vi "Homing v2.vi"(7 "Robot In":i32, 8 "error in":errorcluster, 9 "ToolInsertionOffset":dbl=-54.76, 10 "ToolType":i32=6, 11 "FPGA VI Reference In":refnum<k20>) -> (0 "error out":errorcluster, 1 "Last Stage Posit":dbl[](array[numeric]), 2 "Last Joint Posit":dbl[](array[numeric]), 3 "FPGA VI Reference Out":refnum<k20>)   [LabVIEW 2016]
uses:
  Subsystems/Global Variables.vi
  <vilib>/platform/TimedLoop/XDataNode/XDataNode.xnode
  <vilib>/Platform/TimedLoop/XDataNode/timing_clust.ctl
  <vilib>/Platform/TimedLoop/XDataNode/XDNodeRunTimeDep.lvlib
  <vilib>/Platform/TimedLoop/XDataNode/wakeup.ctl
  <vilib>/Platform/TimedLoop/XDataNode/nitl_modes.ctl
  <vilib>/rvi/interface/nirviReadWriteControl/nirviReadWriteControl.xnode
  Library/KevinLibraryAll/labview2011/kevLib2011.lvlib
  Library/mjglib/var_OCTzHomeDir.vi
  Functions/EyeRobotDLL.dll
  FPGA Bitfiles/PhantomControlPI_FPGATarget_QuadCtr2_E2412E44.lvbitx
  IRISS_FPGA_IO.vi
  NiFpgaLv.dll
  <vilib>/Utility/error.llb/Error Cluster From Error Code.vi
  <vilib>/rvi/errors/niLvFpgaAdjustHostInterfaceError.vi
panel:
  out "Grasp":dbl
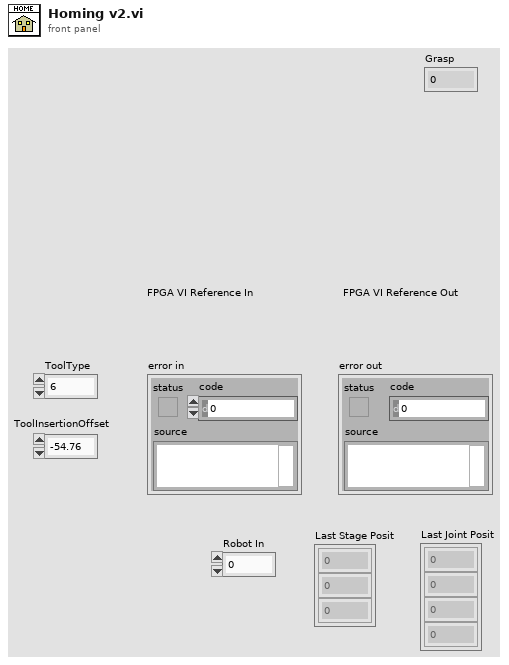
[diagram p1: front panel]
types:
  T1 = typedef "XDNodeRunTimeDep.lvlib/timing_clust.ctl" = cluster{"Expected End [f-1]":u64, "Actual End [f-1]":u64, "Finished Late? [f-1]":bool, "Expected End [i-1]":u64, "Actual End [i-1]":u64, "Finished Late? [i-1]":bool, "Expected Start [i]":u64, "Actual Start [i]":u64, "Expected Start [f]":u64, "Actual Start [f]":u64, "Source Name":string, "Structure Name":string, "Period":i64, "Deadline":i64, "Offset":i64, "Start":i64, "Priority":i32, "Timeout":i32, "Mode":T2, "Wakeup Reason":T3, "Error":errorcluster, "Source Type":string, "Secondary Source Type":string, "Global End Time":u64, "Global Start Time":u64, "Frame Duration":u64, "Iteration Duration":u64, "Assigned CPU":i32, "I/O Scan Engine Mode":u32}
  T2 = typedef "XDNodeRunTimeDep.lvlib/nitl_modes.ctl" = enum32{"No Change", "Process missed periods, maintain original phase", "Discard missed periods, maintain original phase", "Process missed periods, ignore original phase", "Discard missed periods, ignore original phase"}
  T3 = typedef "XDNodeRunTimeDep.lvlib/wakeup.ctl" = enum32{"Normal", "Aborted", "Asynchronous wakeup", "Timing source error", "Timed loop error", "Timeout"}
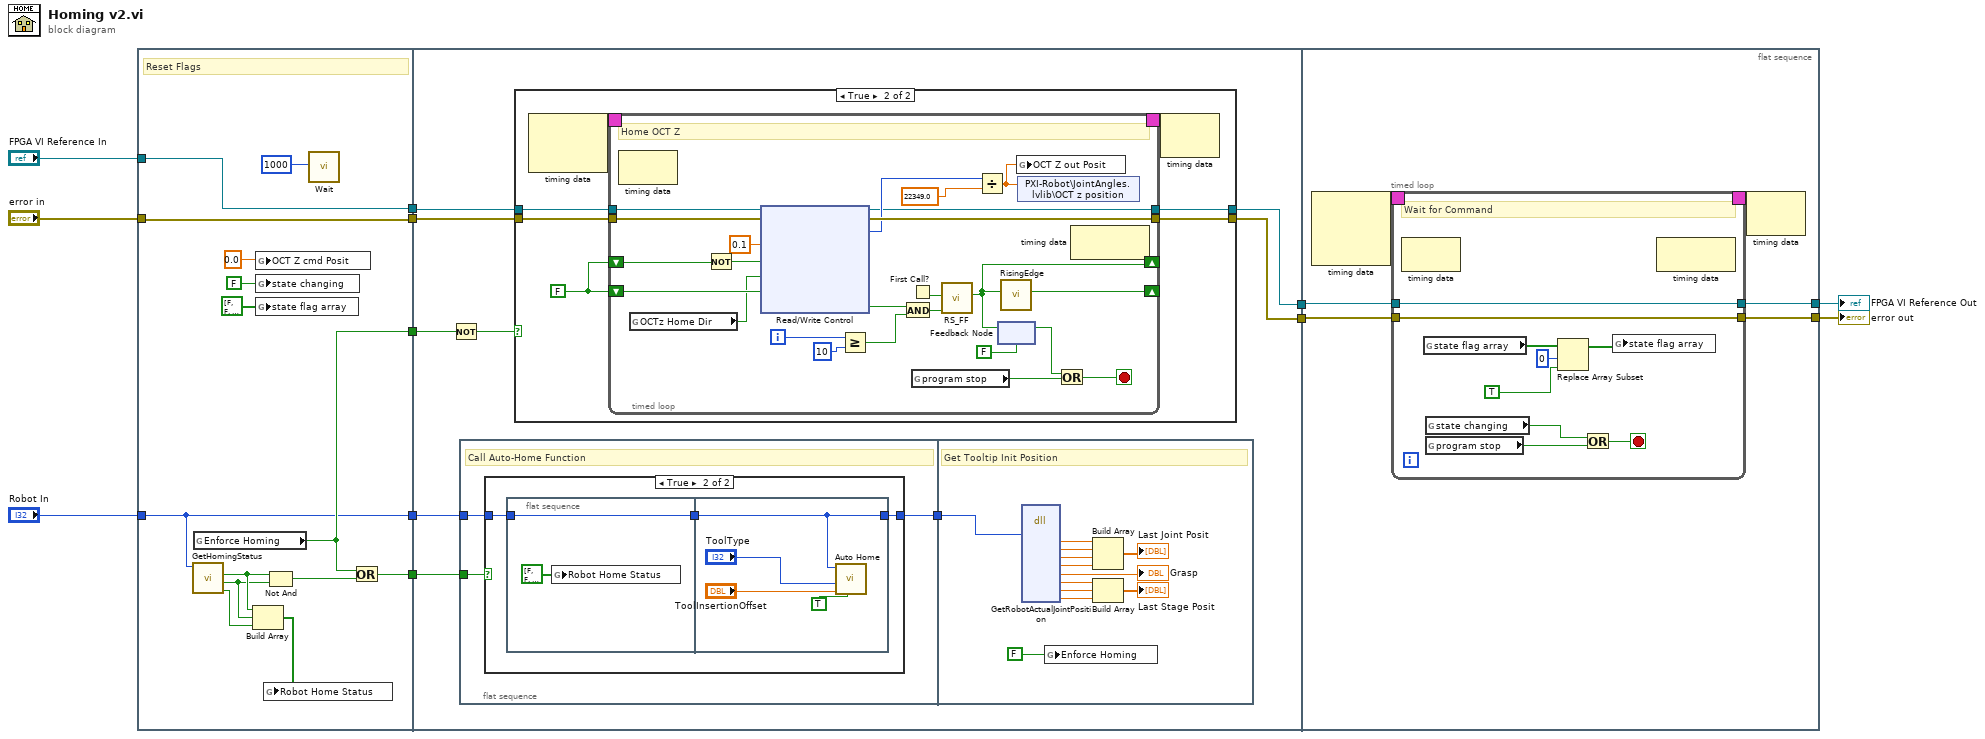
[diagram p0: block diagram]
diagram:
  n1 = flat-sequence {
    tunnel: "FPGA VI Reference In" -> [w26]
    tunnel: "error in" -> [w25]
    tunnel: [w26] -> w8
    tunnel: [w25] -> w7
    tunnel: [w22] -> w5
    tunnel: [w24] -> w3
    tunnel: [w23] -> w2
    tunnel: "Robot In" -> [w22]
    tunnel: w8 -> [w33]
    tunnel: w7 -> [w32]
    tunnel: [w34] -> w6
    tunnel: w5 -> [w31]
    tunnel: [w35] -> w4
    tunnel: w3 -> [w30]
    tunnel: w2 -> [w29]
    tunnel: [w103] -> w10
    tunnel: [w102] -> w9
    tunnel: w6 -> [w100]
    tunnel: w4 -> [w101]
    frame #0 {
      # "Reset Flags"
      n2 = call "GetHomingStatus.vi"("ArmID"=w22) -> ("Homing XYZ Stage Done"=w14:bool, "Homing Tool Done"=w15:bool, "Homing Arm Done"=w16:bool)  [unwired: 4 in]
      n3 = global read "Global Variables.vi" "Enforce Homing"() -> (w23:bool)
      n4 = Build Array(w16, w15, w14) -> (w17:bool[])
      n5 = global write "Global Variables.vi" "OCT Z cmd Posit"(0.0) -> ()
      n6 = global write "Global Variables.vi" "state changing"(FALSE ("state changing")) -> ()
      n7 = global write "Global Variables.vi" "state flag array"(bool[] [FALSE, FALSE, FALSE, FALSE, FALSE, FALSE, FALSE, FALSE, FALSE] ("state flag array")) -> ()
      n8 = global write "Global Variables.vi" "Robot Home Status"(w17) -> ()
      n9 = Not And(1:w15, 2:w16) -> (0:w13:bool)
      n10 = call "Wait"("Count(mSec)"=u32 1000 ("milliseconds to wait")) -> ()  [unwired: 1 out]
      n11 = Or(x=w23, y=w13) -> (x .or. y?=w24:bool)
    }
    frame #1 {
      n12 = Not(x=w29) -> (.not. x?=w27:bool)
      n13 = flat-sequence {
        tunnel: [w36] -> w28
        tunnel: w31 -> [w38]
        tunnel: w30 -> [w37]
        tunnel: w28 -> [w60]
        frame #0 {
          # "Call Auto-Home Function"
          n14 = case shown="True" w37 {
            tunnel: w38 -> [w39 w42]
            tunnel: [w39 w40] -> w36
            frame False {
            }
            frame True {
              n15 = flat-sequence {
                tunnel: w42 -> [w44]
                tunnel: [w44] -> w41
                tunnel: w41 -> [w47]
                tunnel: [w47] -> w40
                frame #0 {
                  n16 = global write "Global Variables.vi" "Robot Home Status"(bool[] [FALSE, FALSE, FALSE, FALSE, FALSE, FALSE, FALSE, FALSE, FALSE] ("state flag array")) -> ()
                }
                frame #1 {
                  n17 = call "Auto Home.vi"(6:TRUE ("Set Tool Type"), 8:"ToolInsertionOffset", 9:"ToolType", "ToolType"=w47) -> ()  [unwired: 8 in]
                }
              }
            }
          }
        }
        frame #1 {
          # "Get Tooltip Init Position"
          n18 = dll-call lib="D:/Kevin/IRISS V2 dev/Host Demo/Functions/EyeRobotDLL.dll" fn="GetRobotActualJointPosition"("armID"=w60) -> ("j0"=w53:dbl, "j1"=w54:dbl, "j2"=w55:dbl, "j3"=w56:dbl, "j4"=→"Grasp":dbl, "j5"=w58:dbl, "j6"=w59:dbl, "j7"=w52:dbl)  [unwired: 13 in, 2 out]
          n19 = global write "Global Variables.vi" "Enforce Homing"(FALSE ("Enforce Homing")) -> ()
          n20 = Build Array(w53, w54, w55, w56) -> (→"Last Joint Posit":dbl[])
          n21 = Build Array(w58, w59, w52) -> (→"Last Stage Posit":dbl[])
        }
      }
      n22 = case shown="True" w27 {
        tunnel: [w62 w67] -> w35
        tunnel: [w61 w66] -> w34
        tunnel: w33 -> [w62 w65]
        tunnel: w32 -> [w61 w64]
        frame False {
        }
        frame True {
          w63 = FALSE ("Rising Edge")
          n23 = node-c288() -> (w69:T1)  [unwired: 2 in]
          n24 = timed-loop {
            timing: w69 -> [_]
            timing-out: [_] -> w68
            tunnel: w65 -> [w90]
            tunnel: w64 -> [w89]
            tunnel: [w72] -> w67
            tunnel: [w88] -> w66
            shift-right: [w85] -> _
            shift-left: w63 -> [w87]
            shift-right: [w81] -> _
            shift-left: w63 -> [w79]
            i -> [w91]
            stop <- w70 stop-if-true
            # "Home OCT Z"
            n25 = node-c288() -> ()  [unwired: 1 in, 1 out]
            n26 = global read "var_OCTzHomeDir.vi" "OCTz Home Dir"() -> (w73:bool)
            n27 = Not(x=w79) -> (.not. x?=w78:bool)
            n28 = xnode "Read/Write Control"("FPGA VI Reference In"=w90, "error in"=w89, "OCT Mot DC"=0.1 ("y"), "INHB OCT Mot"=w78, "DIR OCT Mot"=w73, "Reset 14"=w87) -> ("FPGA VI Reference Out"=w72:refnum<k20>, "error out"=w88:errorcluster, "32 bit Position 14"=w76:i32, "Home OCT z"=w86:bool)
            n29 = Greater Or Equal?(x=w91, y=10) -> (x >= y?=w93:bool)
            n30 = And(x=w86, y=w93) -> (x .and. y?=w83:bool)
            n31 = First Call?() -> (First Call?: T/F=w84:bool)
            n32 = global read "Global Variables.vi" "program stop"() -> (w71:bool)
            n33 = call "RS_FF.vi"("Set"=w83, "Reset"=w84) -> ("Result"=w81:bool)  [unwired: 9 in]
            n34 = Divide(x=w76, y=22349.0) -> (x/y=w74:dbl)
            n35 = feedback #1(FALSE) -> (w80:bool)
            n36 = feedback-in #1(w81) -> ()
            n37 = call "RisingEdge.vi"("Signal In"=w81) -> ("Rising Edge"=w85:bool)  [unwired: 10 in]
            n38 = global write "Global Variables.vi" "OCT Z out Posit"(w74) -> ()
            n39 = shared-variable "PXI-Robot\\JointAngles.lvlib\\OCT z position"(w74) -> ()  [unwired: 1 in, 1 out]
            n40 = Or(x=w80, y=w71) -> (x .or. y?=w70:bool)
            n41 = node-c288() -> ()  [unwired: 1 in, 1 out]
          }
          n42 = node-c288(w68) -> ()  [unwired: 1 out]
        }
      }
    }
    frame #2 {
      n43 = node-c288() -> (w99:T1)  [unwired: 3 in]
      n44 = timed-loop {
        timing: w99 -> [_]
        timing-out: [_] -> w98
        tunnel: w101 -> [w106]
        tunnel: [w106] -> w103
        tunnel: [w105] -> w102
        tunnel: w100 -> [w105]
        stop <- w107 stop-if-true
        # "Wait for Command"
        n45 = node-c288() -> ()  [unwired: 1 in, 1 out]
        n46 = global read "Global Variables.vi" "state flag array"() -> (w111:bool[])
        n47 = global read "Global Variables.vi" "state changing"() -> (w112:bool)
        n48 = global read "Global Variables.vi" "program stop"() -> (w104:bool)
        n49 = Replace Array Subset(array=w111, new element=TRUE ("new element/subarray"), index=0) -> (w110:bool[])
        n50 = Or(x=w112, y=w104) -> (x .or. y?=w107:bool)
        n51 = global write "Global Variables.vi" "state flag array"(w110) -> ()
        n52 = node-c288() -> ()  [unwired: 1 in, 1 out]
      }
      n53 = node-c288(w98) -> ()  [unwired: 1 out]
    }
  }
  "FPGA VI Reference Out" <- w10
  "error out" <- w9
